vi "Pixel_Scan_Engine.vi"(0 "Pixel Scan Parameters In":T1={"Scan Start Pixel"=1, "Scan End Pixel"=1, "Pixel Start Value (-1 to 1)"=-0.5, "Pixel End Value (-1 to 1)"=0.5, "Number of Steps"=0.1}, 2 "Action":T2(ring), 11 "Initial Pixel Values (-1 to 1)":dbl[](array[numeric])) -> ()   [LabVIEW 2014]
uses:
  Pixel Scan Parameters.ctl
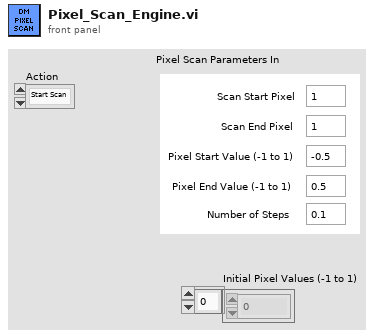
[diagram p1: front panel]
types:
  T1 = typedef "Pixel Scan Parameters.ctl" = cluster{"Scan Start Pixel":i32, "Scan End Pixel":i32, "Pixel Start Value (-1 to 1)":dbl, "Pixel End Value (-1 to 1)":dbl, "Number of Steps":dbl}
  T2 = enum16{"Start Scan", "Reset Counter", "Write DM", "Get Image", "Update Count", "Exit"}
  T3 = enum16{"Reset Counter", "Update Counter", "Get Count"}
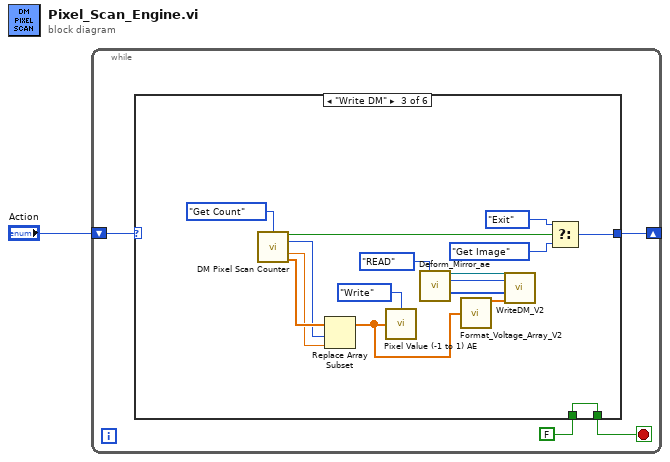
[diagram p0: block diagram]
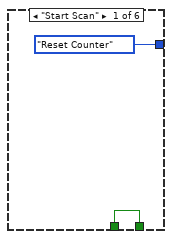
[diagram p2: hidden frame]
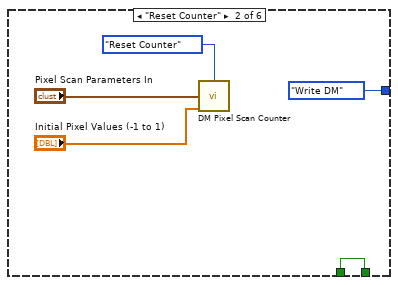
[diagram p3: hidden frame]
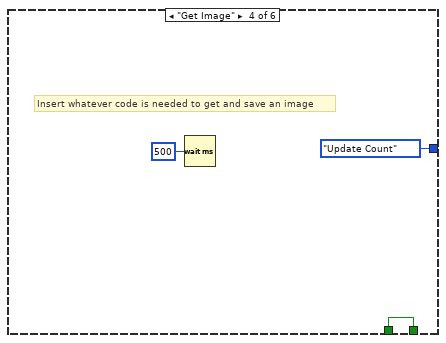
[diagram p4: hidden frame]
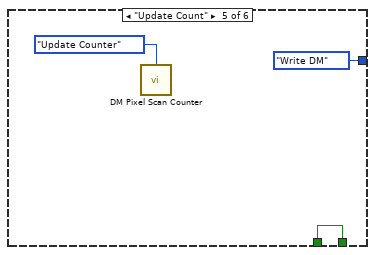
[diagram p5: hidden frame]
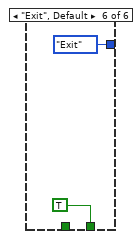
[diagram p6: hidden frame]
diagram:
  n1 = while {
    shift-right: [w2] -> _
    shift-left: "Action" -> [w5]
    stop <- w4 stop-if-true
    n2 = case shown="\"Write DM\"" w5 {
      tunnel: [w7 w8 w14 w31 w32 TRUE] -> w4
      tunnel: FALSE -> [w7 w8 w14 w31 w32 _]
      tunnel: [T2."Reset Counter" ("Action") T2."Write DM" ("Action") w15 T2."Update Count" ("Action") T2."Write DM" ("Action") T2."Exit" ("Action")] -> w2
      frame "Start Scan" {
      }
      frame "Reset Counter" {
        n3 = call "DM Pixel Scan Counter.vi"("Action"=T3."Reset Counter", "Pixel Scan Parameters In"="Pixel Scan Parameters In", "Initial Pixel Values (-1 to 1)"="Initial Pixel Values (-1 to 1)") -> ()  [unwired: 9 in, 4 out]
      }
      frame "Write DM" {
        n4 = call "DM Pixel Scan Counter.vi"("Action"=T3."Get Count") -> ("Scan Done"=w17:bool, "DM Pixel"=w25:i32, "Normalized DM Pixel Value"=w23:dbl, "Initial Pixel Values OUT"=w26:dbl[])  [unwired: 11 in]
        n5 = Replace Array Subset(array=w26, new element=w23, index=w25) -> (w24:dbl[])
        n6 = call "Pixel Value (-1 to 1) AE.vi"("Action"=enum16{"Read", "Write"}."Write", "Pixel Value (-1 to 1)"=w24) -> ()  [unwired: 13 in, 1 out]
        n7 = call "Deform_Mirror_ae.vi"("Enum"=enum16{"WRITE", "READ"}."READ") -> ("Refnum Out"=w18:refnum<k7>, "IDs Out"=w19:i32, "Multi Map Data Out"=w20:i32[])  [unwired: 10 in, 2 out]
        n8 = call "Format_Voltage_Array_V2.vi"("Pixel Level (-1 to 1)"=w24) -> ("Voltage Array (Volts)"=w13:dbl[])  [unwired: 13 in, 1 out]
        n9 = call "WriteDM_V2.vi"("reference in"=w18, "nDevId"=w19, "MultiDM  Mapping"=w20, "Voltage Array in"=w13) -> ()  [unwired: 2 in, 2 out]
        n10 = Select(t=T2."Exit" ("Action"), s=w17, f=T2."Get Image" ("Action")) -> (s? t:f=w15:T2)
      }
      frame "Get Image" {
        # "Insert whatever code is needed to get and save an image"
        n11 = Wait (ms)(milliseconds to wait=u32 500) -> ()  [unwired: 1 out]
      }
      frame "Update Count" {
        n12 = call "DM Pixel Scan Counter.vi"("Action"=T3."Update Counter") -> ()  [unwired: 11 in, 4 out]
      }
      frame "Exit", Default {
      }
    }
  }
